vi "Auto Setup Core.vi"(8 "error in (no error)":errorcluster, 11 "IVI_Scope in":refnum<class "IVI_Scope.lvclass">) -> (0 "error out":errorcluster, 3 "IVI_Scope out":refnum<class "IVI_Scope.lvclass">)   [LabVIEW 2016, in "IVI_Scope.lvlib" / "IVI_Scope.lvclass"]
doc: "This VI automatically configures the instrument.\n\nNotes:\n\nNote \n(1) When you call this VI, the oscilloscope senses the input signal and automatically configures many of the instrument settings. The settings no longer match the cache values for the corresponding properties. Therefore, this VI invalidates all property cache values.\n\n(2) This VI is part of the IviScopeAutoSetup [AS] extension group."
uses:
  IVI_Scope.lvclass
  IVI_Scope.lvclass/IVI_Scope.ctl
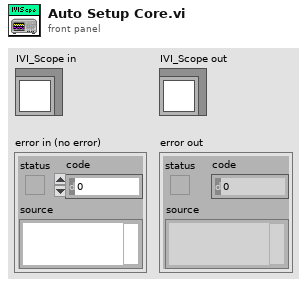
[diagram p1: front panel]
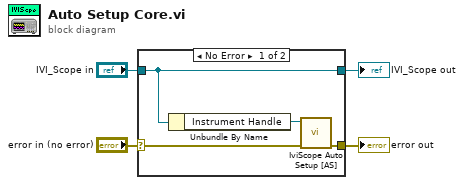
[diagram p0: block diagram]
diagram:
  n1 = case shown="No Error" "error in (no error)" {
    selector: "error in (no error)" -> [w6 w10]
    tunnel: [w5 w10] -> w3
    tunnel: [w8 w9] -> w1
    tunnel: "IVI_Scope in" -> [w8 w9]
    frame No Error {
      n2 = Unbundle By Name(w8) -> ("Instrument Handle"=w7:refnum<k15>)
      n3 = call <vilib>:"IviScope Auto Setup [AS].vi"("error in (no error)"=w6, "instrument handle"=w7) -> ("error out"=w5:errorcluster)  [unwired: 8 in, 1 out]
    }
    frame Error {
    }
  }
  "error out" <- w3
  "IVI_Scope out" <- w1
